vi "Acquire Data from Single Channel2.vi"() -> ()   [LabVIEW 2012]
uses:
  Acquisition Engine/Acquisition Engine State.ctl
  <vilib>/Platform/TimedLoop/XDataNode/timing_clust.ctl
  <vilib>/Platform/TimedLoop/XDataNode/nitl_modes.ctl
  <vilib>/Platform/TimedLoop/XDataNode/wakeup.ctl
  <vilib>/rvi/Emulation/niFpgaSctlEmulationRegisterWithScheduler.vi
  <vilib>/rvi/Emulation/niFpgaSctlEmulationScheduler.vi
  <vilib>/rvi/interface/RandomDataEmulation/nirviRandomDataFPGAFIFO.vi
  <vilib>/rvi/interface/RandomDataEmulation/niFpgaRandomDataHandleErrors.vi
  <vilib>/rvi/eio/common/nirviEmuTemplateMethod_errors.vi
  <vilib>/Platform/TimedLoop/XDataNode/XDataNode.xnode
  <vilib>/rvi/DataTransferAndStorage/Container/XNode/niFpgaContainer.xnode
  <vilib>/rvi/interface/RandomDataEmulation/nirviRandomDataFpgaReadWriteTemplate.vi
  <vilib>/eio/EIONode/EIONode.xnode
  <vilib>/Platform/TimedLoop/XDataNode/XDNodeRunTimeDep.lvlib
panel:
  in  "User Command Commit":bool
  in  "User Command":u8
  out "User Command Idle":bool
  out "User Command Status":u8
  in  "User Data 0":u8
  in  "User Data 1":u8
  out "PLL Locked":bool
  out "Configured?":bool
  in  "Pre Trigger Samples":u16
  in  "Samples per Record":u16=1000
  in  "Load Record Parameters?":bool
  in  "Trigger Hold Off":u16
  in  "Record Count":u16=1
  out "Host Inputs":T1
  in  "Reset?":bool
  in  "Arm Acquisition Engine":bool
  in  "Software Trigger from Host":bool
  in  "Channel":T2(ring)
  out "Host FIFO Time Out":bool
  out "Points Acquired":u64
  out "Current State":T3=enum."Arm Acquisition Engine"
  in  "Trigger Type":T4(ring)=enum."Software Trigger"
  # "Acquisition Parameters I"
  # "User Command Load"
  # "Acquisition Parameters II"
  # "Acquisition Status"
  # "User Command Status"
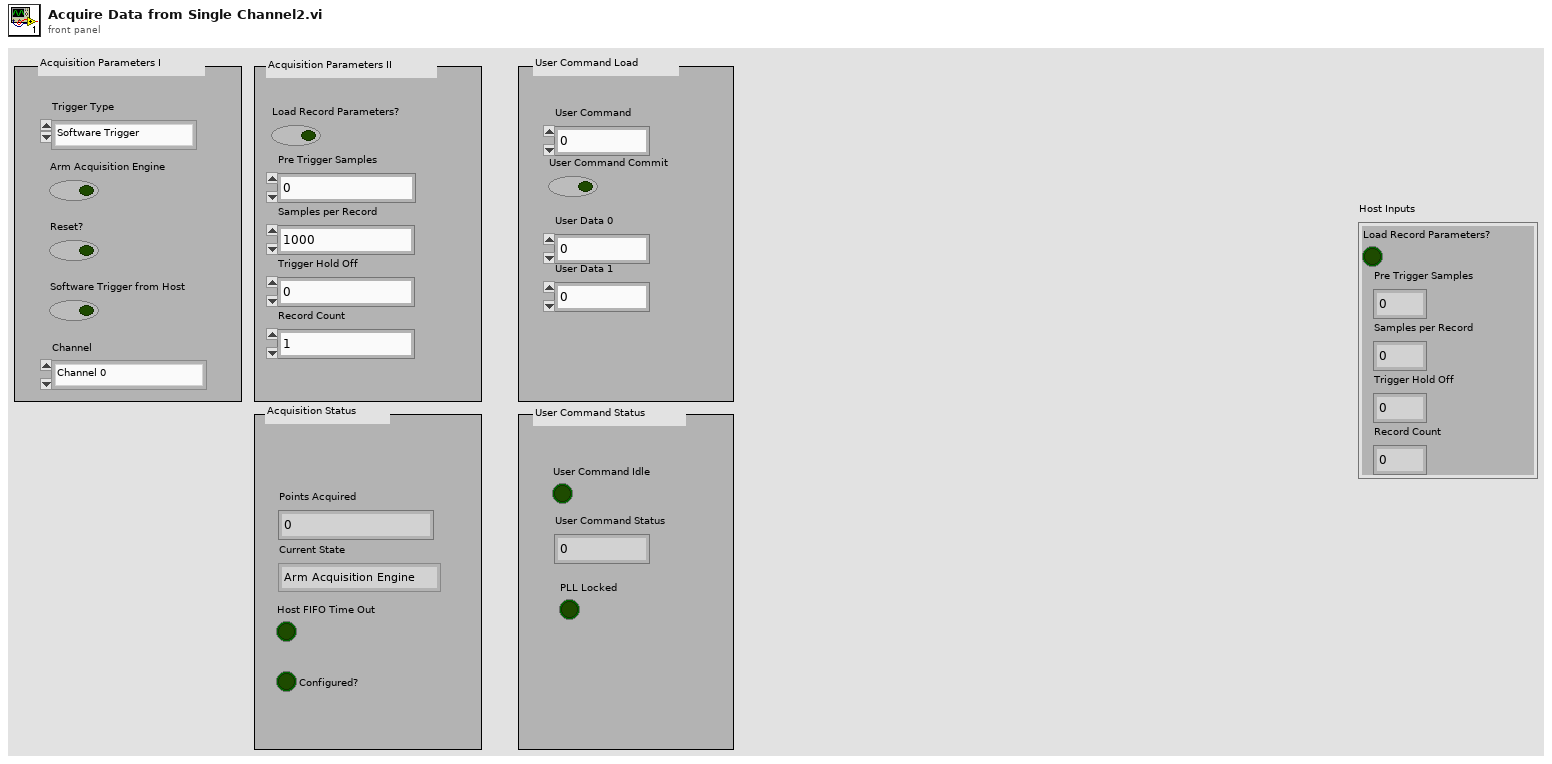
[diagram p1: front panel]
types:
  T1 = cluster{"Load Record Parameters?":bool, "Pre Trigger Samples":u16, "Samples per Record":u16, "Trigger Hold Off":u16, "Record Count":u16}
  T2 = enum16{"Channel 0", "Channel 1", "Channel 2", "Channel 3"}
  T3 = typedef "Acquisition Engine State.ctl" = enum8{"Idle", "Arm Acquisition Engine", "Acquire Pre-Trigger Samples", "Wait for Trigger", "Acquisition Hold Off Time", "Read Data from Buffer", "Check Records Done?", "Re-Arm State", "Flush Available Data"}
  T4 = enum8{"External Digital Trigger", "Software Trigger", "Immediate Trigger"}
  T5 = typedef "XDNodeRunTimeDep.lvlib/timing_clust.ctl" = cluster{"Expected End [f-1]":u64, "Actual End [f-1]":u64, "Finished Late? [f-1]":bool, "Expected End [i-1]":u64, "Actual End [i-1]":u64, "Finished Late? [i-1]":bool, "Expected Start [i]":u64, "Actual Start [i]":u64, "Expected Start [f]":u64, "Actual Start [f]":u64, "Source Name":string, "Structure Name":string, "Period":i64, "Deadline":i64, "Offset":i64, "Start":i64, "Priority":i32, "Timeout":i32, "Mode":T6, "Wakeup Reason":T7, "Error":errorcluster, "Source Type":string, "Secondary Source Type":string, "Global End Time":u64, "Global Start Time":u64, "Frame Duration":u64, "Iteration Duration":u64, "Assigned CPU":i32, "I/O Scan Engine Mode":u32}
  T6 = typedef "XDNodeRunTimeDep.lvlib/nitl_modes.ctl" = enum32{"No Change", "Process missed periods, maintain original phase", "Discard missed periods, maintain original phase", "Process missed periods, ignore original phase", "Discard missed periods, ignore original phase"}
  T7 = typedef "XDNodeRunTimeDep.lvlib/wakeup.ctl" = enum32{"Normal", "Aborted", "Asynchronous wakeup", "Timing source error", "Timed loop error", "Timeout"}
  T8 = typedef "Multi-Channel Analog Input Data.ctl" = i16[]
  T9 = typedef "Acquisition Parameters.ctl" = cluster{"Pre Trigger Samples":u16, "Post-Trigger Samples":u16, "Trigger Hold Off":u16, "Record Count":u16}
  T10 = typedef "Buffer Parameters.ctl" = cluster{"Init Read and Write Pointer":bool, "Write Pointer":u16, "Read Pointer":u16, "Buffer Length-1":u16}
  T11 = typedef "Acquisition Status.ctl" = cluster{"Reset":bool, "Acquisition Engine Start (Arm)":bool, "Current State":T3, "Trig Offset":u8, "Points Unread":u16, "Points Acquired":u16, "Records Done":u16, "Start of Read":bool, "End of Read":bool, "Start of Record":bool, "End of Record":bool, "Ready for Ref Trig":bool, "In Reset?":bool}
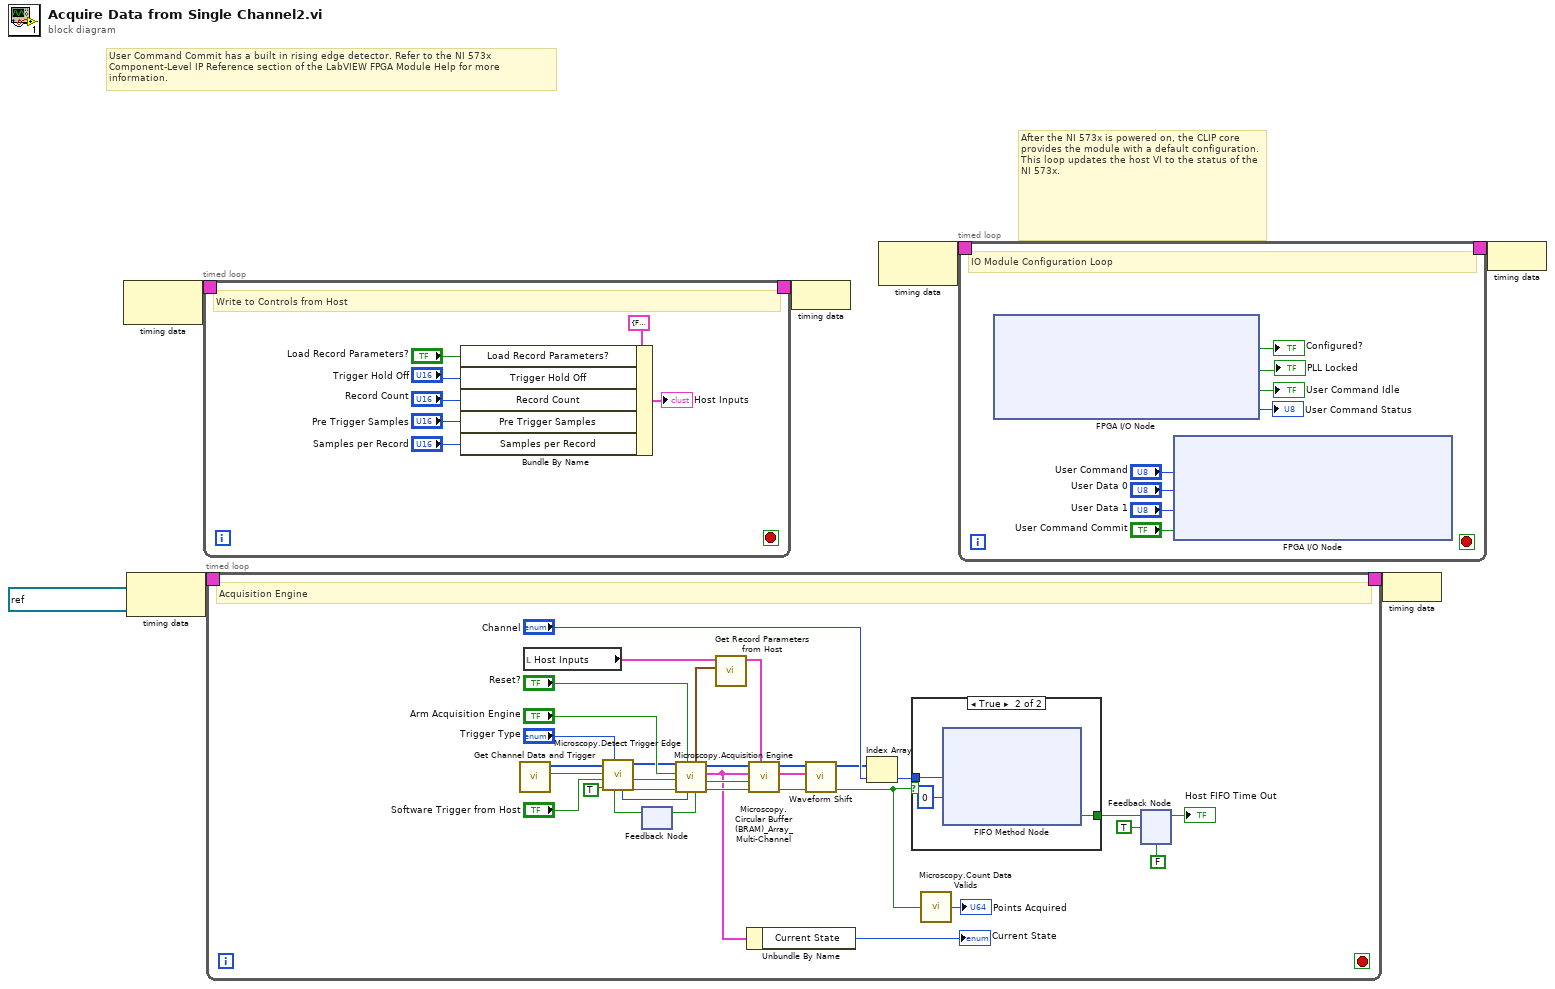
[diagram p0: block diagram]
diagram:
  # "After the NI 573x is powered on, the CLIP core provides the module with a default configuration. This loop updates the host VI to the status of the NI 573x."
  # "User Command Commit has a built in rising edge detector. Refer to the NI 573x Component-Level IP Reference section of the LabVIEW FPGA Module Help for more information."
  n1 = node-c288() -> (w5:T5)  [unwired: 1 in]
  n2 = node-c288(refnum<k21> "IO Module Clock 0" ("Source Name")) -> (w7:T5)
  n3 = timed-loop {
    timing: w5 -> [_]
    timing-out: [_] -> w4
    stop <- _ stop-if-true
    # "Write to Controls from Host"
    n4 = Bundle By Name(cluster=T1 {"Load Record Parameters?"=FALSE, "Pre Trigger Samples"=0, "Samples per Record"=0, "Trigger Hold Off"=0, "Record Count"=0} ("Record Parameters"), "Load Record Parameters?"="Load Record Parameters?", "Trigger Hold Off"="Trigger Hold Off", "Record Count"="Record Count", "Pre Trigger Samples"="Pre Trigger Samples", "Samples per Record"="Samples per Record") -> (→"Host Inputs":T1)
  }
  n5 = timed-loop {
    timing: w7 -> [_]
    timing-out: [_] -> w6
    stop <- _ stop-if-true
    # "Acquisition Engine"
    n6 = call "Get Channel Data and Trigger.vi"() -> ("Trigger"=w26:bool, "Data"=w36:i16[])  [unwired: 10 in]
    n7 = local read "Host Inputs"() -> (w23:T1)
    n8 = feedback #1() -> (w29:bool)  [unwired: 1 in]
    n9 = call "Microscopy.Detect Trigger Edge.vi"("Ready for Next Record?"=w29, "Trigger Type"="Trigger Type", "Data Valid In"=TRUE, "Software Trigger from Host"="Software Trigger from Host", "Digita IO Trigger"=w26, "Analog Channel Data"=w36) -> ("Data Valid Out"=w42:bool, "Reference Trigger Edge?"=w43:bool, "Analog Channel Data"=w44:T8, "Trig Offset"=w17:u8)  [unwired: 2 in]
    n10 = call "Get Record Parameters from Host.vi"("Record Parameters"=w23) -> ("Acquisition Parameters"=w39:T9, "Buffer Parameters"=w38:T10)  [unwired: 9 in]
    n11 = call "Microscopy.Acquisition Engine.vi"("Acquisition Parameters"=w39, "Trig Offset"=w17, "Reset?"="Reset?", "Data Valid In"=w42, "Reference Trigger Edge?"=w43, "Arm Acquisition Engine"="Arm Acquisition Engine", "Channel Data In"=w44) -> ("Data Valid Out"=w45:bool, "Read from Buffer"=w46:bool, "Acquisition Status"=w28:T11, "Channel Data Out"=w47:T8, "Ready for Ref Trig"=w30:bool)
    n12 = feedback-in #1(w30) -> ()
    n13 = Unbundle By Name(w28) -> ("Current State"=→"Current State":T3)
    n14 = call "Microscopy.Circular Buffer (BRAM)_Array_Multi-Channel.vi"("Buffer Pointers"=w38, "Input Valid"=w45, "Read Data?"=w46, "Acquisition Status In"=w28, "Input Write Data"=w47) -> ("Output Valid"=w19:bool, "Acquisition Status Out"=w21:T11, "Output Write Data"=w22:T8)  [unwired: 4 in]
    n15 = call "Waveform Shift.vi"("Input Data Valid"=w19, "Acquisition Status In"=w21, "Input Data"=w22) -> ("Output Data Valid"=w18:bool, "Output Data"=w20:i16[])  [unwired: 6 in, 1 out]
    n16 = Index Array(array=w20, index="Channel") -> (element=w24:i16)
    n17 = case shown="True" w18 {
      tunnel: w24 -> [_ w52]
      tunnel: [_ w50] -> w35
      frame False {
      }
      frame True {
        n18 = xnode ("FIFO Method Node")("Element"=w52, "Timeout"=0) -> ("Timed Out?"=w50:bool)  [unwired: 1 in, 1 out]
      }
    }
    n19 = call "Microscopy.Count Data Valids.vi"("Data Valid"=w18) -> ("Counter"=→"Points Acquired":u64)  [unwired: 14 in]
    n20 = feedback-in #2(w35, TRUE) -> ()
    n21 = feedback #2(FALSE ("Timed Out?")) -> (→"Host FIFO Time Out":bool)
  }
  n22 = node-c288(w4) -> ()
  n23 = node-c288() -> (w2:T5)  [unwired: 1 in]
  n24 = timed-loop {
    timing: w2 -> [_]
    timing-out: [_] -> w1
    stop <- _ stop-if-true
    # "IO Module Configuration Loop"
    n25 = xnode "FPGA I/O Node"() -> ("IO Module\\Initialization Done"=→"Configured?":bool, "IO Module\\PLL Locked"=→"PLL Locked":bool, "IO Module\\User Command Idle"=→"User Command Idle":bool, "IO Module\\User Command Status"=→"User Command Status":u8)  [unwired: 4 in, 4 out]
    n26 = xnode ("FPGA I/O Node")("IO Module\\User Command"="User Command", "IO Module\\User Data 0"="User Data 0", "IO Module\\User Data 1"="User Data 1", "IO Module\\User Command Commit"="User Command Commit") -> ()  [unwired: 4 in, 4 out]
  }
  n27 = node-c288(w6) -> ()
  n28 = node-c288(w1) -> ()
